vi "LibXML_ConcatenateTrees.vi"(8 "error in":errorcluster, 9 "XML-tree2":T1[](array[typedef]), 11 "XML-tree1":T1[](array[typedef])) -> (0 "error out":errorcluster, 3 "XML-tree out":T1[](array[typedef]))   [LabVIEW 2019, in "Tools.lvlib" / "LibXML.lvlib"]
uses:
  LibXML.lvlib
  LibXML_Element.ctl
  LibXML_Attribute.ctl
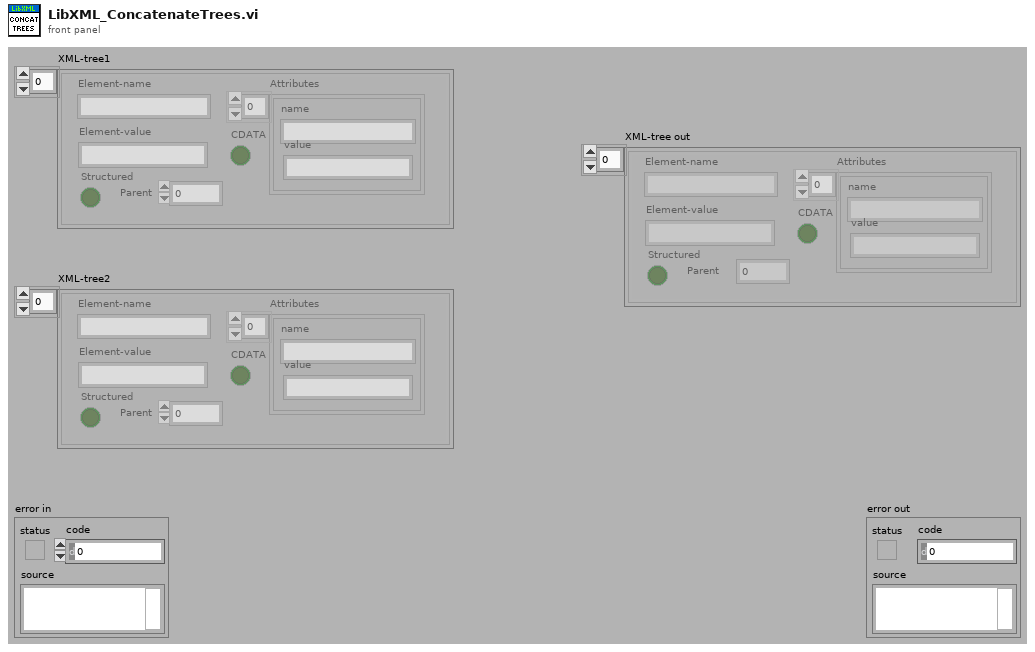
[diagram p1: front panel]
types:
  T1 = typedef "Tools.lvlib/LibXML.lvlib/LibXML_Element.ctl" = cluster{"Element-name":string, "Attributes":T2[], "Element-value":string, "CDATA":bool, "Parent":i32, "Structured":bool}
  T2 = typedef "Tools.lvlib/LibXML.lvlib/LibXML_Attribute.ctl" = cluster{"name":string, "value":string}
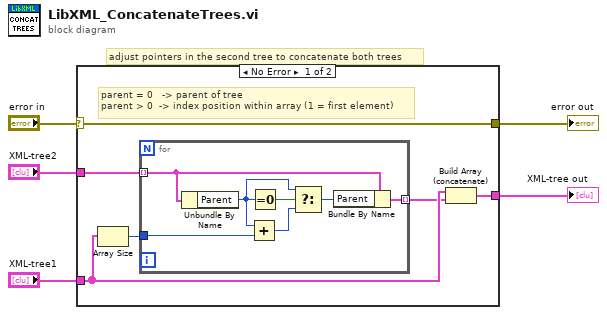
[diagram p0: block diagram]
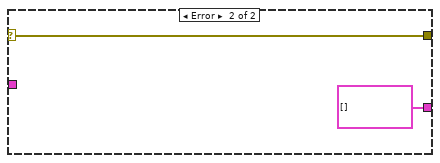
[diagram p2: hidden frame]
diagram:
  # "adjust pointers in the second tree to concatenate both trees"
  n1 = case shown="No Error" "error in" {
    selector: "error in" -> [w6 w20]
    tunnel: "XML-tree2" -> [w11 _]
    tunnel: "XML-tree1" -> [w10 _]
    tunnel: [w7 T1[] []] -> w3
    tunnel: [w6 w20] -> w1
    frame No Error {
      # "parent = 0   -> parent of tree\nparent > 0  -> index position within array (1 = first element)"
      n2 = Array Size(array=w10) -> (size(s)=w9:i32)
      n3 = for {
        tunnel: w11 -> [w18] mode=indexing
        tunnel: w9 -> [w17]
        tunnel: [w12] -> w8 mode=indexing
        n4 = Unbundle By Name(w18) -> ("Parent"=w14:i32)
        n5 = Add(x=w14, y=w17) -> (x+y=w15:i32)
        n6 = Equal To 0?(x=w14) -> (x = 0?=w16:bool)
        n7 = Select(t=w14, s=w16, f=w15) -> (s? t:f=w13:i32)
        n8 = Bundle By Name(cluster=w18, "Parent"=w13) -> (w12:T1)
      }
      n9 = Build Array (concatenate)(w10, w8) -> (w7:T1[])
    }
    frame Error {
    }
  }
  "XML-tree out" <- w3
  "error out" <- w1
